vi "Timestamp Month Difference.vi"(1 "Time Stamp 2":timestamp, 2 "Time Stamp":timestamp) -> (0 "Month Difference":i32)   [LabVIEW 2020]
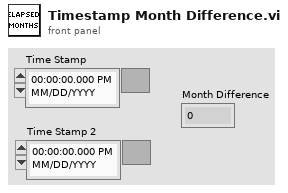
[diagram p1: front panel]
types:
  T1 = typedef "LVDateTimeRec.ctl" = cluster{"fractional second":dbl, "second":i32, "minute":i32, "hour":i32, "day of month":i32, "month":i32, "year":i32, "day of week":i32, "day of year":i32, "DST":i32}
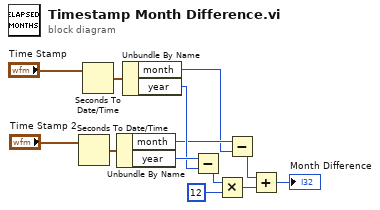
[diagram p0: block diagram]
diagram:
  n1 = Seconds To Date/Time(time stamp (now)="Time Stamp 2") -> (date time rec=w11:T1)  [unwired: 1 in]
  n2 = Seconds To Date/Time(time stamp (now)="Time Stamp") -> (date time rec=w10:T1)  [unwired: 1 in]
  n3 = Unbundle By Name(w11) -> ("month"=w4:i32, "year"=w9:i32)
  n4 = Unbundle By Name(w10) -> ("month"=w3:i32, "year"=w8:i32)
  n5 = Subtract(x=w9, y=w8) -> (x-y=w7:i32)
  n6 = Multiply(x=w7, y=12) -> (x*y=w5:i32)
  n7 = Subtract(x=w4, y=w3) -> (x-y=w2:i32)
  n8 = Add(x=w2, y=w5) -> (x+y=→"Month Difference":i32)
